vi "ModbusCRC.vi"(11 "ModbusCRCSettings":T1={"DataFIFO"="InclinometerRxCRCFIFO", "CalculateFIFO"="InclinometerCalculateCRCFIFO", "CRCFIFO"="InclinometerCalculatedCRCFIFO"}) -> ()   [LabVIEW 2016]
uses:
  ModbusCRCSettings.ctl
  ModbusCRCData.ctl
  ModbusCRCStates.ctl
  <vilib>/Platform/TimedLoop/XDataNode/timing_clust.ctl
  <vilib>/Platform/TimedLoop/XDataNode/nitl_modes.ctl
  <vilib>/Platform/TimedLoop/XDataNode/wakeup.ctl
  <vilib>/rvi/Emulation/niFpgaSctlEmulationGetInTimedLoop.vi
  <vilib>/rvi/Emulation/niFpgaEmulationReportErrorSimple.vi
  <vilib>/rvi/Emulation/niFpgaGetClockAttributes.vi
  <vilib>/rvi/Emulation/niFpgaCriticalErrorInLSC.vi
  <vilib>/rvi/DataTransferAndStorage/Container/Common/niFpgaContainerExecOnDevCompGetState.vi
  <vilib>/rvi/Emulation/niFpgaEmulationIsFPGAContextNoSignature.vi
  <vilib>/rvi/errors/niFpgaSetErrorForExecOnDevCompSimple.vi
  <vilib>/rvi/eio/common/nirviEmuReportErrorAndStop.vi
  <vilib>/rvi/DataTransferAndStorage/Container/Common/niFpgaContainerGetUniqueNameForEmu.vi
  <vilib>/rvi/FIFO/Fifo_Resource/nirvififoEmulationSetSize.vi
  <vilib>/rvi/FIFO/Fifo_Resource/nirviFifoEmulationQueueMgr.vi
  <instcachedir>/0/nirviFifoEmulationQueueMgr_E5CAEC123FF24DC58D834DCA3CDAA9B5.lvgen/nirviFifoEmulationQueueMgr_E5CAEC123FF24DC58D834DCA3CDAA9B5_009.vi
  <vilib>/rvi/FIFO/Fifo_Resource/nirvififoEmulationDetermineInputValidOut.vi
  <vilib>/rvi/FIFO/Fifo_Resource/nirvififoEmulationCreateLock.vi
  <vilib>/rvi/Emulation/niFpgaProcessEmulError.vi
  <vilib>/rvi/FIFO/Fifo_Resource/nirvififoEmulationObtainLock.vi
  <vilib>/rvi/FIFO/Fifo_Resource/nirvififoEmulationReleaseLock.vi
  <vilib>/rvi/occurrence/nirviWaitOnOccurrenceBase.vi
  <vilib>/rvi/errors/nirviReportUnexpectedCaseInternalError.vi
  <vilib>/rvi/errors/nirviReportUnexpectedCaseInternalError (U32).vi
  <vilib>/Utility/error.llb/Clear Errors.vi
  <vilib>/rvi/interface/RandomDataEmulation/niFpgaRandomDataHandleErrors.vi
  <instcachedir>/0/nirviFifoEmulationQueueMgr_E5CAEC123FF24DC58D834DCA3CDAA9B5.lvgen/nirviFifoEmulationQueueMgr_E5CAEC123FF24DC58D834DCA3CDAA9B5_004.vi
  <instcachedir>/0/nirviFifoEmulationQueueMgr_E5CAEC123FF24DC58D834DCA3CDAA9B5.lvgen/nirviFifoEmulationQueueMgr_E5CAEC123FF24DC58D834DCA3CDAA9B5_002.vi
  <vilib>/Platform/TimedLoop/XDataNode/XDataNode.xnode
  <vilib>/rvi/DataTransferAndStorage/Container/XNode/niFpgaContainer.xnode
  <vilib>/rvi/FIFO/Fifo_Resource/niFpgaFifoEmulationRefIn.vi
  <vilib>/Platform/TimedLoop/XDataNode/XDNodeRunTimeDep.lvlib
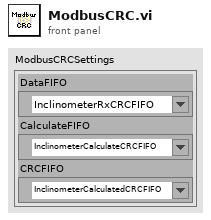
[diagram p1: front panel]
types:
  T1 = typedef "ModbusCRCSettings.ctl" = cluster{"DataFIFO":refnum<k21>, "CalculateFIFO":refnum<k21>, "CRCFIFO":refnum<k21>}
  T2 = typedef "ModbusCRCData.ctl" = cluster{"State":T3, "Bit":u8, "CRC":u16}
  T3 = typedef "ModbusCRCStates.ctl" = enum16{"WaitForData", "ProcessData", "CheckForPublish", "PublishCRC"}
  T4 = typedef "XDNodeRunTimeDep.lvlib/timing_clust.ctl" = cluster{"Expected End [f-1]":u64, "Actual End [f-1]":u64, "Finished Late? [f-1]":bool, "Expected End [i-1]":u64, "Actual End [i-1]":u64, "Finished Late? [i-1]":bool, "Expected Start [i]":u64, "Actual Start [i]":u64, "Expected Start [f]":u64, "Actual Start [f]":u64, "Source Name":string, "Structure Name":string, "Period":i64, "Deadline":i64, "Offset":i64, "Start":i64, "Priority":i32, "Timeout":i32, "Mode":T5, "Wakeup Reason":T6, "Error":errorcluster, "Source Type":string, "Secondary Source Type":string, "Global End Time":u64, "Global Start Time":u64, "Frame Duration":u64, "Iteration Duration":u64, "Assigned CPU":i32, "I/O Scan Engine Mode":u32}
  T5 = typedef "XDNodeRunTimeDep.lvlib/nitl_modes.ctl" = enum32{"No Change", "Process missed periods, maintain original phase", "Discard missed periods, maintain original phase", "Process missed periods, ignore original phase", "Discard missed periods, ignore original phase"}
  T6 = typedef "XDNodeRunTimeDep.lvlib/wakeup.ctl" = enum32{"Normal", "Aborted", "Asynchronous wakeup", "Timing source error", "Timed loop error", "Timeout"}
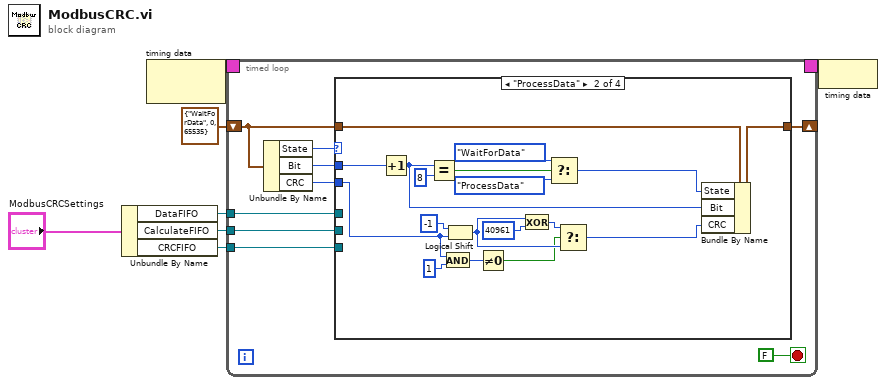
[diagram p0: block diagram]
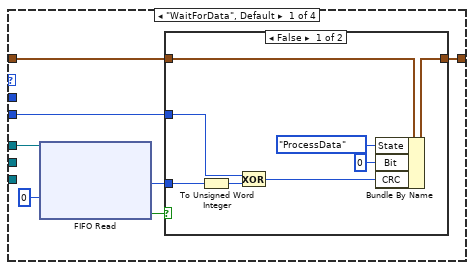
[diagram p2: hidden frame]
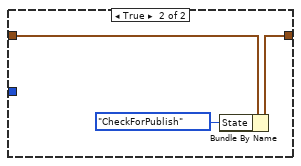
[diagram p3: hidden frame]
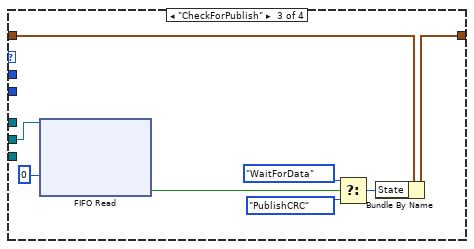
[diagram p4: hidden frame]
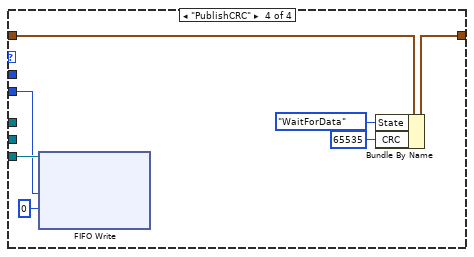
[diagram p5: hidden frame]
diagram:
  n1 = Unbundle By Name("ModbusCRCSettings") -> ("DataFIFO"=w3:refnum<k21>, "CalculateFIFO"=w2:refnum<k21>, "CRCFIFO"=w1:refnum<k21>)
  n2 = node-c288() -> (w6:T4)  [unwired: 1 in]
  n3 = timed-loop {
    shift-right: [w15] -> _
    shift-left: T2 {"State"=enum."WaitForData", "Bit"=0, "CRC"=65535} ("ModbusCRCData") -> [w14]
    timing: w6 -> [_]
    timing-out: [_] -> w5
    tunnel: w3 -> [w12]
    tunnel: w2 -> [w11]
    tunnel: w1 -> [w10]
    stop <- FALSE stop-if-true
    n4 = Unbundle By Name(w14) -> ("State"=w16:T3, "Bit"=w9:u8, "CRC"=w13:u16)
    n5 = case shown="\"ProcessData\"" w16 {
      tunnel: [w18 w51 w59 w66] -> w15
      tunnel: w14 -> [w23 w52 w60 w67]
      tunnel: w13 -> [w17 w36 _ w63]
      tunnel: w12 -> [w22 _ _ _]
      tunnel: w11 -> [_ _ w58 _]
      tunnel: w10 -> [_ _ _ w64]
      tunnel: w9 -> [_ w50 _ _]
      frame "WaitForData", Default {
        n6 = xnode ("FIFO Read")("Timeout"=0, "FIFO In"=w22) -> ("Element"=w19:u8, "Timed Out?"=w20:bool)  [unwired: 1 out]
        n7 = case shown="False" w20 {
          tunnel: w23 -> [w31 w34]
          tunnel: w19 -> [w28 _]
          tunnel: [w30 w33] -> w18
          tunnel: w17 -> [w26 _]
          frame False {
            n8 = To Unsigned Word Integer(number=w28) -> (unsigned 16bit integer=w27:u16)
            n9 = Exclusive Or(1:w27, 2:w26) -> (0:w25:u16)
            n10 = Bundle By Name(cluster=w31, "State"=ModbusCRCStates."ProcessData", "Bit"=u8 0, "CRC"=w25) -> (w30:T2)
          }
          frame True {
            n11 = Bundle By Name(cluster=w34, "State"=ModbusCRCStates."CheckForPublish") -> (w33:T2)
          }
        }
      }
      frame "ProcessData" {
        n12 = Increment(x=w50) -> (x+1=w44:u8)
        n13 = Equal?(x=w44, y=u8 8) -> (x = y?=w48:bool)
        n14 = And(x=w36, y=u16 1) -> (x .and. y?=w37:u16)
        n15 = Logical Shift(y=i16 -1, x=w36) -> (x << y=w43:u16)
        n16 = Not Equal To 0?(x=w37) -> (x != 0?=w38:bool)
        n17 = Exclusive Or(1:u16 40961 ("y"), 2:w43) -> (0:w42:u16)
        n18 = Select(t=ModbusCRCStates."WaitForData", s=w48, f=ModbusCRCStates."ProcessData" ("State")) -> (s? t:f=w45:T3)
        n19 = Select(t=w42, s=w38, f=w43) -> (s? t:f=w35:u16)
        n20 = Bundle By Name(cluster=w52, "State"=w45, "Bit"=w44, "CRC"=w35) -> (w51:T2)
      }
      frame "CheckForPublish" {
        n21 = xnode ("FIFO Read")("Timeout"=0, "FIFO In"=w58) -> ("Timed Out?"=w56:bool)  [unwired: 2 out]
        n22 = Select(t=ModbusCRCStates."WaitForData" ("State"), s=w56, f=ModbusCRCStates."PublishCRC" ("State")) -> (s? t:f=w53:T3)
        n23 = Bundle By Name(cluster=w60, "State"=w53) -> (w59:T2)
      }
      frame "PublishCRC" {
        n24 = xnode ("FIFO Write")("Element"=w63, "Timeout"=0, "FIFO In"=w64) -> ()  [unwired: 2 out]
        n25 = Bundle By Name(cluster=w67, "State"=ModbusCRCStates."WaitForData", "CRC"=u16 65535) -> (w66:T2)
      }
    }
  }
  n26 = node-c288(w5) -> ()
